vi "ReadDigitalInterface_old.vi"(7 "error in":errorcluster, 9 "ON/OFF":bool, 10 "VISA resource name in":refnum<visa-resource-name>) -> (0 "error out":errorcluster, 2 "Extend Device Status":T1, 3 "VISA resource name out":refnum<visa-resource-name>)   [LabVIEW 2014]
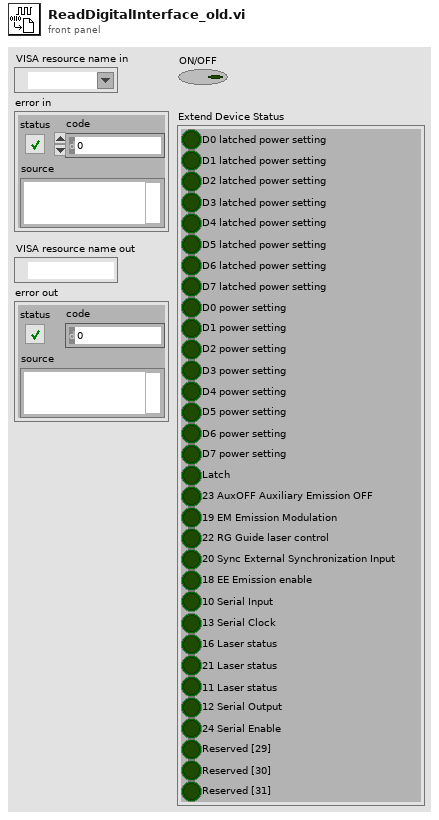
[diagram p1: front panel]
types:
  T1 = cluster{"D0 latched power setting":bool, "D1 latched power setting":bool, "D2 latched power setting":bool, "D3 latched power setting":bool, "D4 latched power setting":bool, "D5 latched power setting":bool, "D6 latched power setting":bool, "D7 latched power setting":bool, "D0 power setting":bool, "D1 power setting":bool, "D2 power setting":bool, "D3 power setting":bool, "D4 power setting":bool, "D5 power setting":bool, "D6 power setting":bool, "D7 power setting":bool, "Latch":bool, "23 AuxOFF Auxiliary Emission OFF":bool, "19 EM Emission Modulation":bool, "22 RG Guide laser control":bool, "20 Sync External Synchronization Input":bool, "18 EE Emission enable":bool, "10 Serial Input":bool, "13 Serial Clock":bool, "16 Laser status":bool, "21 Laser status":bool, "11 Laser status":bool, "12 Serial Output":bool, "24 Serial Enable":bool, "Reserved [29]":bool, "Reserved [30]":bool, "Reserved [31]":bool}
  T2 = cluster{"Boolean array[0]":bool, "Boolean array[1]":bool, "Boolean array[2]":bool, "Boolean array[3]":bool, "Boolean array[4]":bool, "Boolean array[5]":bool, "Boolean array[6]":bool, "Boolean array[7]":bool, "Boolean array[8]":bool, "Boolean array[9]":bool, "Boolean array[10]":bool, "Boolean array[11]":bool, "Boolean array[12]":bool, "Boolean array[13]":bool, "Boolean array[14]":bool, "Boolean array[15]":bool, "Boolean array[16]":bool, "Boolean array[17]":bool, "Boolean array[18]":bool, "Boolean array[19]":bool, "Boolean array[20]":bool, "Boolean array[21]":bool, "Boolean array[22]":bool, "Boolean array[23]":bool, "Boolean array[24]":bool, "Boolean array[25]":bool, "Boolean array[26]":bool, "Boolean array[27]":bool, "Boolean array[28]":bool, "Boolean array[29]":bool, "Boolean array[30]":bool, "Boolean array[31]":bool}
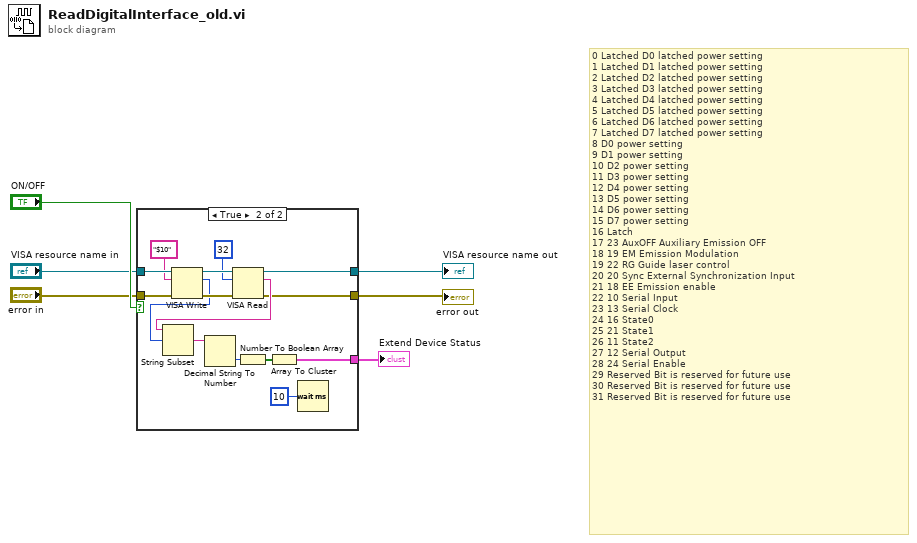
[diagram p0: block diagram]
diagram:
  # "0 Latched D0 latched power setting\n1 Latched D1 latched power setting\n2 Latched D2 latched power setting\n3 Latched D3 latched power setting\n4 Latched D4 latched power setting\n5 Latched D5 latched power setting\n6 Latched D6 latched power setting\n7 Latched D7 latched power setting\n8 D0 power setting\n9 D1 power setting\n10 D2 power setting\n11 D3 power setting\n12 D4 power setting\n13 D5 power setting\n14 D6 power setting\n15 D7 power setting\n16 Latch\n17 23 AuxOFF Auxiliary Emission OFF\n18 19 EM Emission Modulation\n19 22 RG Guide laser control\n20 20 Sync External Synchronization Input\n21 18 EE Emission enable\n22 10 Serial Input\n23 13 Serial Clock\n24 16 State0\n25 21 State1\n26 11 State2\n27 12 Serial Output\n28 24 Serial Enable\n29 Reserved Bit is reserved for future use\n30 Reserved Bit is reserved for future use\n31 Reserved Bit is reserved for future use"
  n1 = case shown="True" "ON/OFF" {
    tunnel: "VISA resource name in" -> [w8 w21]
    tunnel: "error in" -> [w7 w20]
    tunnel: [w8 w10] -> w3
    tunnel: [w7 w9] -> w2
    tunnel: [_ w13] -> w1
    frame False {
    }
    frame True {
      n2 = VISA Write(VISA resource name=w21, write buffer="$10", error in (no error)=w20) -> (VISA resource name out=w22:refnum<visa-resource-name>, return count=w15:u32, error out=w23:errorcluster)
      n3 = VISA Read(VISA resource name=w22, byte count=u32 32, error in (no error)=w23) -> (VISA resource name out=w10:refnum<visa-resource-name>, read buffer=w16:string, error out=w9:errorcluster)  [unwired: 1 out]
      n4 = String Subset(string=w16, offset (0)=w15) -> (substring=w17:string)  [unwired: 1 in]
      n5 = Decimal String To Number(string=w17) -> (number=w18:i32)  [unwired: 2 in, 1 out]
      n6 = Number To Boolean Array(number=w18) -> (Boolean array=w14:bool[])
      n7 = Array To Cluster(array=w14) -> (cluster=w13:T2)
      n8 = Wait (ms)(milliseconds to wait=u32 10) -> ()  [unwired: 1 out]
    }
  }
  "Extend Device Status" <- w1
  "VISA resource name out" <- w3
  "error out" <- w2
